vi "GetQ_array enum.vi"(8 "error in (no error)":errorcluster, 10 "Array Enums":variant) -> (0 "error out":errorcluster, 1 "foundArray":bool[](array[boolean]), 2 "QueueArray":refnum<queue>[](array[refnum]))   [LabVIEW 2020, in "QDict.lvlib"]
doc: "Developed by Kevin Thompson\nkevin@thompsonengineering.net\n\nCopyright 2021\nThompson Engineering, LLC"
uses:
  QDict.lvlib
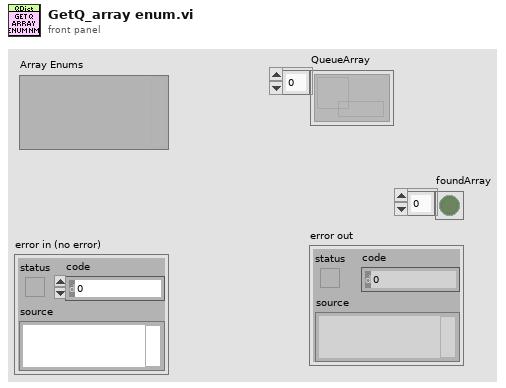
[diagram p1: front panel]
types:
  T1 = typedef "Type Descriptor Enumeration__ogtk.ctl" = enum8{"<Null>", "I8", "I16", "I32", "I64", "U8", "U16", "U32", "U64", "SGL", "DBL", "EXT", "CSG", "CDB", "CXT", "0x0F", "0x10", "0x11", "0x12", "0x13", "0x14", "Enum U8", "Enum U16", "Enum U32", "Enum U64", "SGL PQ", "DBL PQ", "EXT PQ", "CSG PQ", "CDB PQ", "CXT PQ", "0x1F", "0x20", "Boolean", "0x22", "0x23", "0x24", "0x25", "0x26", "0x27", "0x28", "0x29", "0x2A", "0x2B", "0x2C", "0x2D", "0x2E", "0x2F", "String", "0x31", "Path", "Pict", "0x34", "0x35", "0x36", "DAQ", "0x38", "0x39", "0x3A", "0x3B", "0x3C", "0x3D", "0x3E", "0x3F", "Array", "0x41", "0x42", "0x43", "0x44", "0x45", "0x46", "0x47", "0x48", "0x49", "0x4A", "0x4B", "0x4C", "0x4D", "0x4E", "0x4F", "Cluster", "0x51", "0x52", "Variant", "Waveform", "0x55", "0x56", "0x57", "0x58", "0x59", "0x5A", "0x5B", "0x5C", "0x5D", "0x5E", "0x5F", "0x60", "0x61", "0x62", "0x63", "0x64", "0x65", "0x66", "0x67", "0x68", "0x69", "0x6A", "0x6B", "0x6C", "0x6D", "0x6E", "0x6F", "Refnum"}
  T2 = typedef "TD Dynamic CVT DVR--ref.ctl" = refnum<data-value>
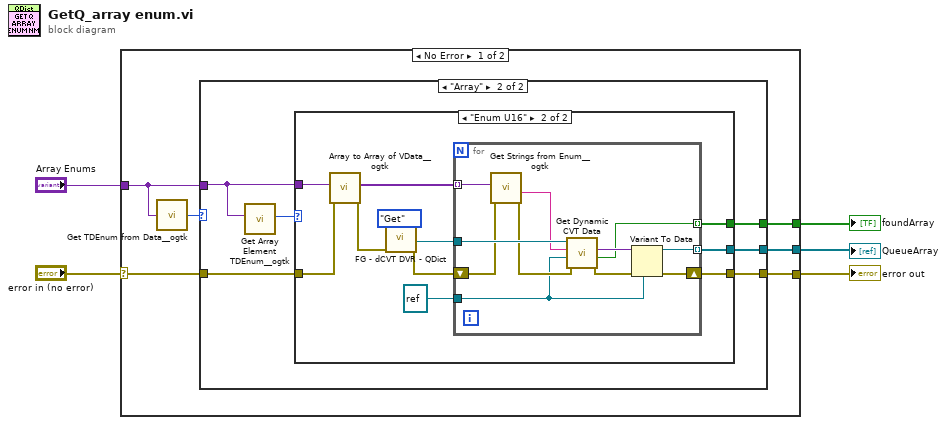
[diagram p0: block diagram]
diagram:
  n1 = case shown="No Error" "error in (no error)" {
    selector: "error in (no error)" -> [w11 w42]
    tunnel: [w9 w42] -> w5
    tunnel: "Array Enums" -> [w6 _]
    tunnel: [w10 _] -> w3
    tunnel: [w8 _] -> w2
    frame No Error {
      n2 = call <userlib>:"Get TDEnum from Data__ogtk.vi"("Data"=w6) -> ("Type Descriptor Enumeration"=w7:T1)  [unwired: 4 in]
      n3 = case shown="\"Array\"" w7 {
        tunnel: w11 -> [w12 w18]
        tunnel: [_ w17] -> w10
        tunnel: [w12 w16] -> w9
        tunnel: [_ w15] -> w8
        tunnel: w6 -> [_ w13]
        frame "<Null>", Default {
        }
        frame "Array" {
          n4 = call <userlib>:"Get Array Element TDEnum__ogtk.vi"("Array"=w13) -> ("Element Type"=w14:T1)  [unwired: 9 in, 1 out]
          n5 = case shown="\"Enum U16\"" w14 {
            tunnel: w18 -> [w19 w21]
            tunnel: [_ w26] -> w17
            tunnel: [w19 w25] -> w16
            tunnel: [_ w24] -> w15
            tunnel: w13 -> [_ w23]
            frame "<Null>", Default {
            }
            frame "Enum U16" {
              n6 = call <userlib>:"Array to Array of VData__ogtk.vi"("error in (no error)"=w21, "MultiD Array"=w23) -> ("error out"=w20:errorcluster, "1D Array of Variants"=w22:variant[])  [unwired: 8 in]
              n7 = call "FG - dCVT DVR - QDict.vi"("error in (no error)"=w20, "Action (Get)"=enum16{"Init", "Get", "Set"}."Get") -> ("dCVT QMH out"=w29:T2, "error out"=w28:errorcluster)  [unwired: 7 in]
              n8 = for {
                tunnel: w29 -> [w41]
                tunnel: refnum<queue> refnum ("queue out") -> [w31]
                tunnel: [w38] -> w26 mode=indexing
                tunnel: [w36] -> w24 mode=indexing
                shift-right: [w37] -> w25
                shift-left: w28 -> [w33]
                tunnel: w22 -> [w35] mode=indexing
                n9 = call <userlib>:"Get Strings from Enum__ogtk.vi"("error in (no error)"=w33, "Enum"=w35) -> ("error out"=w32:errorcluster, "String Value"=w34:string)  [unwired: 6 in, 2 out]
                n10 = call <vilib>:"Get Dynamic CVT Data.vi"("error in (no error)"=w32, "default value (empty variant)"=w31, "DataName"=w34, "dCVT DVR"=w41) -> ("error out"=w40:errorcluster, "found"=w36:bool, "value"=w39:variant)  [unwired: 4 in, 1 out]
                n11 = Variant To Data(error in=w40, type=w31, Variant=w39) -> (data=w38:refnum<queue>, error out=w37:errorcluster)
              }
            }
          }
        }
      }
    }
    frame Error {
    }
  }
  "error out" <- w5
  "QueueArray" <- w3
  "foundArray" <- w2
